vi "STRING LENGTH.vi"() -> ()   [LabVIEW 2019]
panel:
  out "STRING LENTH":i32
  in  "STRING":string="HE IS A BOY"
  # "STRING LENGTH"
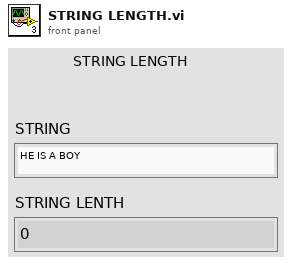
[diagram p1: front panel]
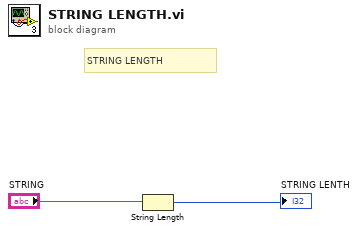
[diagram p0: block diagram]
diagram:
  # "STRING LENGTH"
  n1 = String Length(string="STRING") -> (length=→"STRING LENTH":i32)
